vi "New Graph.vi"(0 "Process_REF":string="Temperature", 1 "Waveform":waveform(dbl)) -> ()   [LabVIEW 2018]
uses:
  <vilib>/Waveform/WDTOps.llb/WDT Append Waveforms DBL.vi
panel:
  out "Waveform Graph":waveform(dbl)[](graph)
  out "error out":errorcluster
  in  "error in (no error)":errorcluster
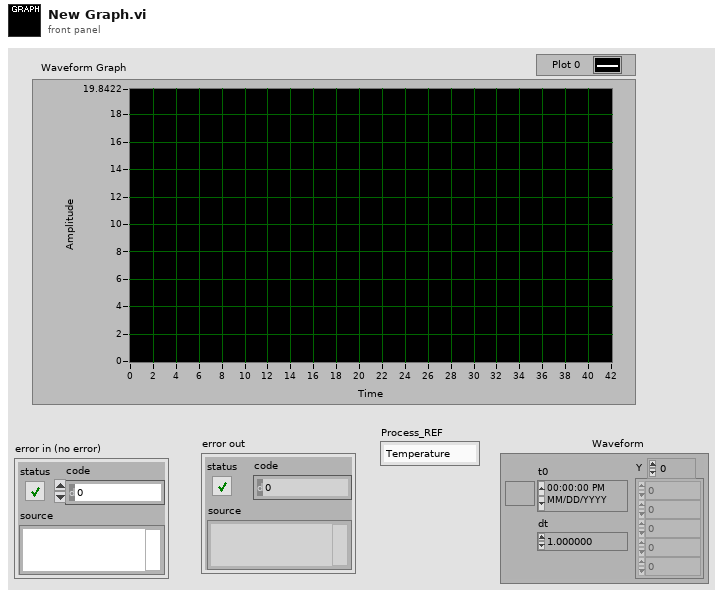
[diagram p1: front panel]
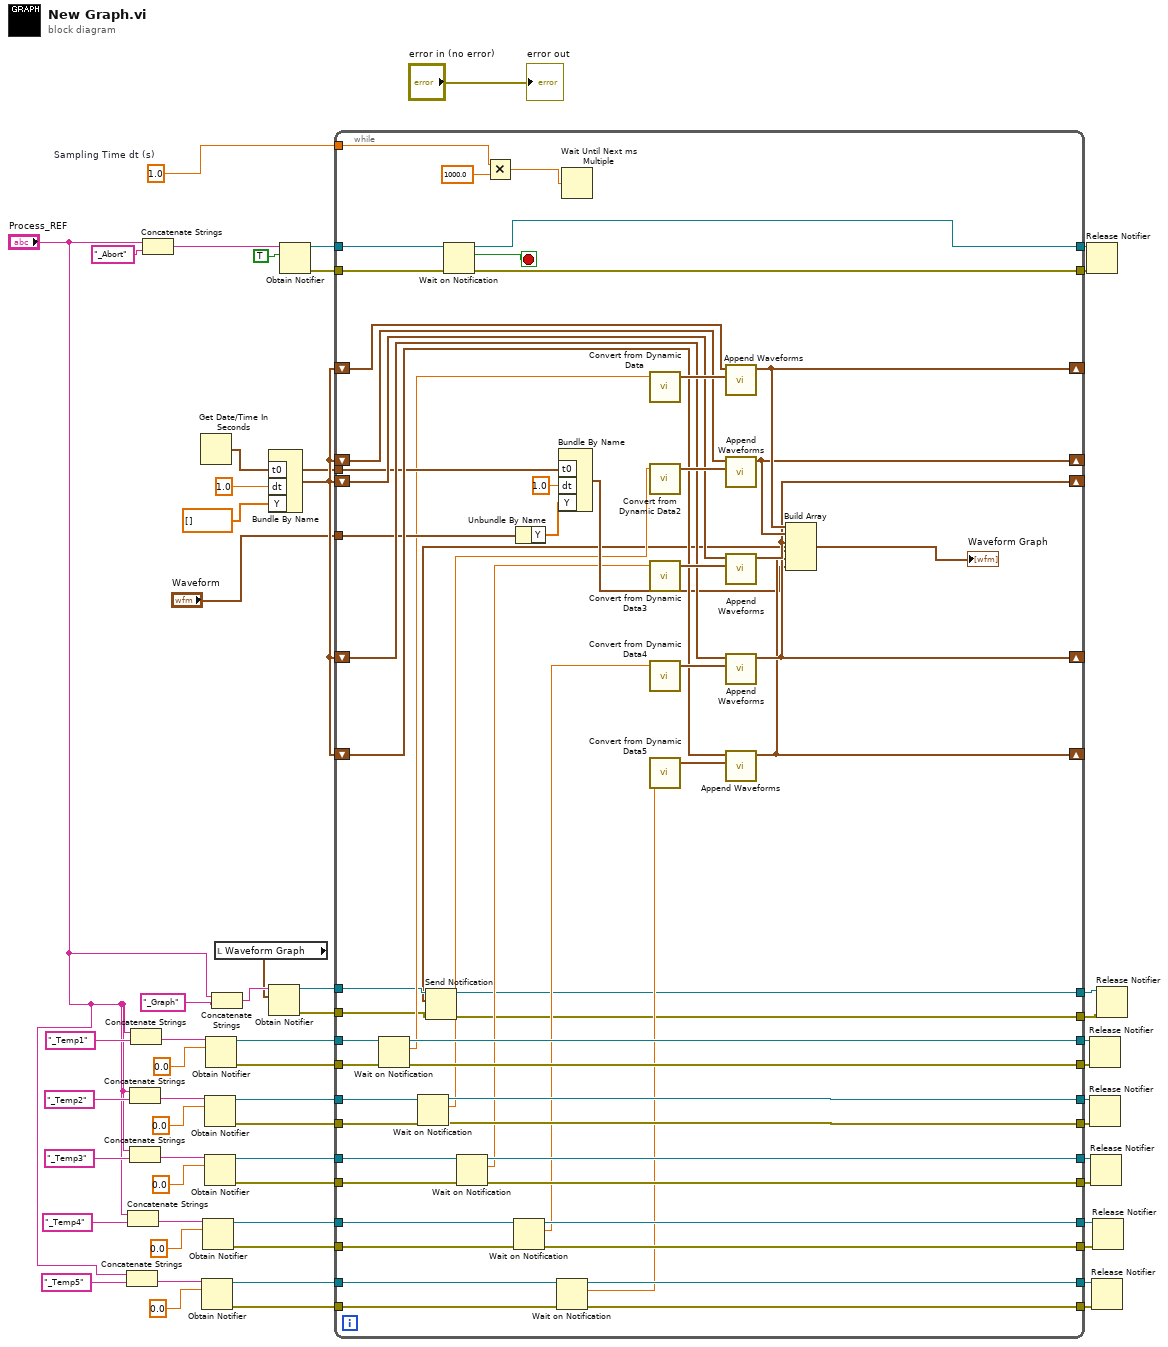
[diagram p0: block diagram]
diagram:
  w9 = 1.0  # Sampling Time dt (s)
  n1 = Concatenate Strings("Process_REF", "_Temp5") -> (w29:string)
  n2 = Concatenate Strings("Process_REF", "_Temp4") -> (w32:string)
  n3 = Concatenate Strings("Process_REF", "_Temp2") -> (w38:string)
  n4 = Concatenate Strings("Process_REF", "_Temp3") -> (w35:string)
  n5 = Concatenate Strings("Process_REF", "_Temp1") -> (w45:string)
  n6 = Concatenate Strings("Process_REF", "_Abort") -> (w51:string)
  n7 = Get Date/Time In Seconds() -> (seconds since 1Jan1904=w11:timestamp)
  n8 = Obtain Notifier(name (unnamed)=w29, notification data type=0.0) -> (notifier out=w24:refnum<notifier>, error out=w21:errorcluster)  [unwired: 2 in, 1 out]
  n9 = Obtain Notifier(name (unnamed)=w32, notification data type=0.0) -> (notifier out=w25:refnum<notifier>, error out=w20:errorcluster)  [unwired: 2 in, 1 out]
  n10 = Obtain Notifier(name (unnamed)=w38, notification data type=0.0) -> (notifier out=w27:refnum<notifier>, error out=w23:errorcluster)  [unwired: 2 in, 1 out]
  n11 = Obtain Notifier(name (unnamed)=w35, notification data type=0.0) -> (notifier out=w26:refnum<notifier>, error out=w22:errorcluster)  [unwired: 2 in, 1 out]
  n12 = Obtain Notifier(name (unnamed)=w45, notification data type=0.0) -> (notifier out=w43:refnum<notifier>, error out=w41:errorcluster)  [unwired: 2 in, 1 out]
  n13 = Concatenate Strings("Process_REF", "_Graph") -> (w4:string)
  n14 = local read "Waveform Graph"() -> (w3:waveform(dbl)[])
  n15 = Bundle By Name("t0"=w11, "dt"=1.0, "Y"=dbl[] []) -> (w47:waveform(dbl))  [unwired: 1 in]
  n16 = Obtain Notifier(name (unnamed)=w4, notification data type=w3) -> (notifier out=w5:refnum<notifier>, error out=w2:errorcluster)  [unwired: 2 in, 1 out]
  n17 = Obtain Notifier(name (unnamed)=w51, notification data type=TRUE) -> (notifier out=w57:refnum<notifier>, error out=w56:errorcluster)  [unwired: 2 in, 1 out]
  n18 = while {
    tunnel: w57 -> [w105]
    tunnel: w56 -> [w102]
    tunnel: [w104] -> w55
    tunnel: [w103] -> w54
    shift-right: [w81] -> _
    shift-left: w47 -> [w110]
    shift-right: [w80] -> _
    shift-left: w47 -> [w109]
    shift-right: [w79] -> _
    shift-left: w47 -> [w108]
    shift-right: [w78] -> _
    shift-left: w47 -> [w107]
    shift-right: [w77] -> _
    shift-left: w47 -> [w106]
    tunnel: [w100] -> w42
    tunnel: w43 -> [w101]
    tunnel: w41 -> [w99]
    tunnel: [w98] -> w40
    tunnel: w27 -> [w95]
    tunnel: w26 -> [w96]
    tunnel: w25 -> [w94]
    tunnel: w24 -> [w97]
    tunnel: [w93] -> w13
    tunnel: w23 -> [w92]
    tunnel: w22 -> [w91]
    tunnel: w21 -> [w90]
    tunnel: w20 -> [w89]
    tunnel: [w88] -> w12
    tunnel: [w87] -> w14
    tunnel: [w86] -> w15
    tunnel: [w85] -> w17
    tunnel: [w84] -> w16
    tunnel: [w83] -> w19
    tunnel: [w82] -> w18
    tunnel: w11 -> [w74]
    tunnel: "Waveform" -> [w72]
    tunnel: w9 -> [w70]
    tunnel: [w62] -> w6
    tunnel: w5 -> [w61]
    tunnel: w2 -> [w60]
    tunnel: [w59] -> w1
    stop <- w64 stop-if-true
    n19 = Wait on Notification(notifier=w101, error in (no error)=w99) -> (notifier out=w100:refnum<notifier>, notification=w63:dbl, error out=w98:errorcluster)  [unwired: 2 in, 1 out]
    n20 = Wait on Notification(notifier=w95, error in (no error)=w92) -> (notifier out=w93:refnum<notifier>, notification=w68:dbl, error out=w88:errorcluster)  [unwired: 2 in, 1 out]
    n21 = Wait on Notification(notifier=w105, error in (no error)=w102) -> (notifier out=w104:refnum<notifier>, notification=w64:bool, error out=w103:errorcluster)  [unwired: 2 in, 1 out]
    n22 = Wait on Notification(notifier=w96, error in (no error)=w91) -> (notifier out=w86:refnum<notifier>, notification=w67:dbl, error out=w87:errorcluster)  [unwired: 2 in, 1 out]
    n23 = Multiply(x=w70, y=1000.0) -> (x*y=w69:dbl)
    n24 = Wait on Notification(notifier=w94, error in (no error)=w89) -> (notifier out=w85:refnum<notifier>, notification=w66:dbl, error out=w84:errorcluster)  [unwired: 2 in, 1 out]
    n25 = Unbundle By Name(w72) -> ("Y"=w75:dbl[])
    n26 = Wait on Notification(notifier=w97, error in (no error)=w90) -> (notifier out=w83:refnum<notifier>, notification=w65:dbl, error out=w82:errorcluster)  [unwired: 2 in, 1 out]
    n27 = Bundle By Name("t0"=w74, "dt"=1.0, "Y"=w75) -> (w73:waveform(dbl))  [unwired: 1 in]
    n28 = Wait Until Next ms Multiple(millisecond multiple=w69) -> ()  [unwired: 1 out]
    n29 = call "Convert from Dynamic Data"("Dynamic Data Type"=w63) -> ("Waveform"=w115:waveform(dbl))  [unwired: 3 in]
    n30 = call "Convert from Dynamic Data2"("Dynamic Data Type"=w68) -> ("Waveform"=w114:waveform(dbl))  [unwired: 3 in]
    n31 = call "Convert from Dynamic Data3"("Dynamic Data Type"=w67) -> ("Waveform"=w113:waveform(dbl))  [unwired: 3 in]
    n32 = call "Convert from Dynamic Data4"("Dynamic Data Type"=w66) -> ("Waveform"=w112:waveform(dbl))  [unwired: 3 in]
    n33 = call "Convert from Dynamic Data5"("Dynamic Data Type"=w65) -> ("Waveform"=w111:waveform(dbl))  [unwired: 3 in]
    n34 = call-poly <vilib>:"Append Waveforms.vi"("waveform B"=w115, "waveform A"=w110) -> ("waveform out"=w81:waveform(dbl))  [unwired: 8 in, 1 out]
    n35 = call-poly <vilib>:"Append Waveforms.vi"("waveform B"=w114, "waveform A"=w109) -> ("waveform out"=w80:waveform(dbl))  [unwired: 8 in, 1 out]
    n36 = call-poly <vilib>:"Append Waveforms.vi"("waveform B"=w113, "waveform A"=w108) -> ("waveform out"=w79:waveform(dbl))  [unwired: 8 in, 1 out]
    n37 = call-poly <vilib>:"Append Waveforms.vi"("waveform B"=w112, "waveform A"=w107) -> ("waveform out"=w78:waveform(dbl))  [unwired: 8 in, 1 out]
    n38 = call-poly <vilib>:"Append Waveforms.vi"("waveform B"=w111, "waveform A"=w106) -> ("waveform out"=w77:waveform(dbl))  [unwired: 8 in, 1 out]
    n39 = Build Array(w81, w80, w79, w78, w77, w73) -> (w58:waveform(dbl)[])
    "Waveform Graph" <- w58
    n40 = Send Notification(notification=w58, notifier=w61, error in (no error)=w60) -> (notifier out=w62:refnum<notifier>, error out=w59:errorcluster)
  }
  n41 = Release Notifier(notifier=w55, error in (no error)=w54) -> ()  [unwired: 1 in, 3 out]
  n42 = Release Notifier(notifier=w42, error in (no error)=w40) -> ()  [unwired: 1 in, 3 out]
  n43 = Release Notifier(notifier=w13, error in (no error)=w12) -> ()  [unwired: 1 in, 3 out]
  n44 = Release Notifier(notifier=w15, error in (no error)=w14) -> ()  [unwired: 1 in, 3 out]
  n45 = Release Notifier(notifier=w19, error in (no error)=w18) -> ()  [unwired: 1 in, 3 out]
  n46 = Release Notifier(notifier=w17, error in (no error)=w16) -> ()  [unwired: 1 in, 3 out]
  n47 = Release Notifier(notifier=w6, error in (no error)=w1) -> ()  [unwired: 1 in, 3 out]
  "error out" <- "error in (no error)"
